vi "RP Read Status VISA.vi"(8 "Error In":errorcluster, 9 "Status offset":u64, 10 "Read config":bool, 11 "VISA resource":refnum<visa-resource-name>) -> (0 "Error Out":errorcluster, 1 "Status response":u32=1 format="0x%x (%d)", 3 "VISA resource out":refnum<visa-resource-name>)   [LabVIEW 2015]
uses:
  RP Command.ctl
  RP Write Command VISA.vi
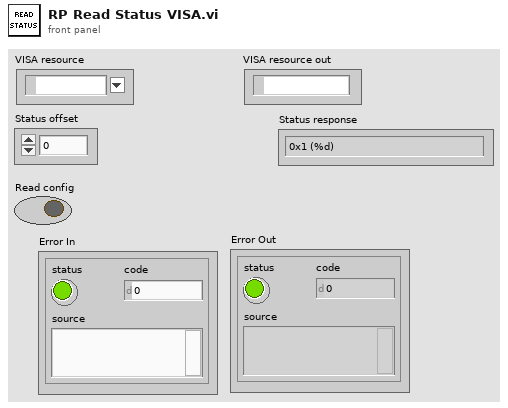
[diagram p1: front panel]
types:
  T1 = typedef "RP Command.ctl" = enum16{"Reset", "Read IDN", "Stop server", "Get status", "Get temperature", "Connect client", "Arm", "Software trigger", "Get whole buffer", "Get chunk", "System call", "Get config", "Set config", "Recieve data", "Play pattern", "Transmit data"}
  T2 = enum16{"big-endian, network order", "native, host order", "little-endian"}
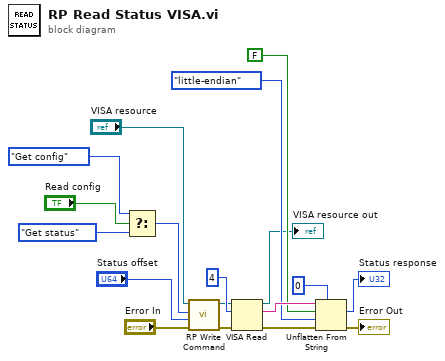
[diagram p0: block diagram]
diagram:
  n1 = Select(t=RP_Command."Get config" ("Command number"), s="Read config", f=RP_Command."Get status" ("Command number")) -> (s? t:f=w3:T1)
  n2 = call-poly "RP Write Command.vi"("Error In"="Error In", "Command payload"="Status offset", "Command number"=w3, "VISA resource"="VISA resource") -> ("Error Out"=w8:errorcluster, "VISA resource out"=w9:refnum<visa-resource-name>)  [unwired: 5 in, 1 out]
  n3 = VISA Read(VISA resource name=w9, byte count=u32 4 ("bytes to read"), error in (no error)=w8) -> (VISA resource name out=→"VISA resource out":refnum<visa-resource-name>, read buffer=w16:string, error out=w14:errorcluster)  [unwired: 1 out]
  n4 = Unflatten From String(type=u32 0, binary string=w16, data includes array or string size? (T)=FALSE, byte order (0:big-endian, network order)=T2."little-endian", error in (no error)=w14) -> (value=→"Status response":u32, error out=→"Error Out":errorcluster)  [unwired: 1 out]
